vi "Test Panel - Sample (SubVI).vi"(8 "error in":errorcluster) -> (0 "error out":errorcluster, 3 "Data Out":T1)   [LabVIEW 2019]
uses:
  Controls/Sample-state.ctl
  <vilib>/httpClient/POSTBuffer.vi
  <vilib>/httpClient/LabVIEWHTTPClient.lvlib
panel:
  in  "Select Specimen From the list:":u16(ring) items=["Please Select..", "1 | 1", "2 | 2", "3 | 3", "4 | 4"]
  in  "Add/Remove Speciment":bool
  in  "Select Existing Job From the list:":u16(ring) items=["Please Select", "Job-001", "Job-002", "Job-003", "10125", "110125", "130125", "MB2695,S2"]
  in  "Refresh Button":bool
  in  "TAB":enum32{"Specimen Details"}(tab)
  in  "Close":bool
  in  "save":bool
  in  "table specimen":string[][](table)
  out "Table job record":string[][](table)
  in  "create new":bool
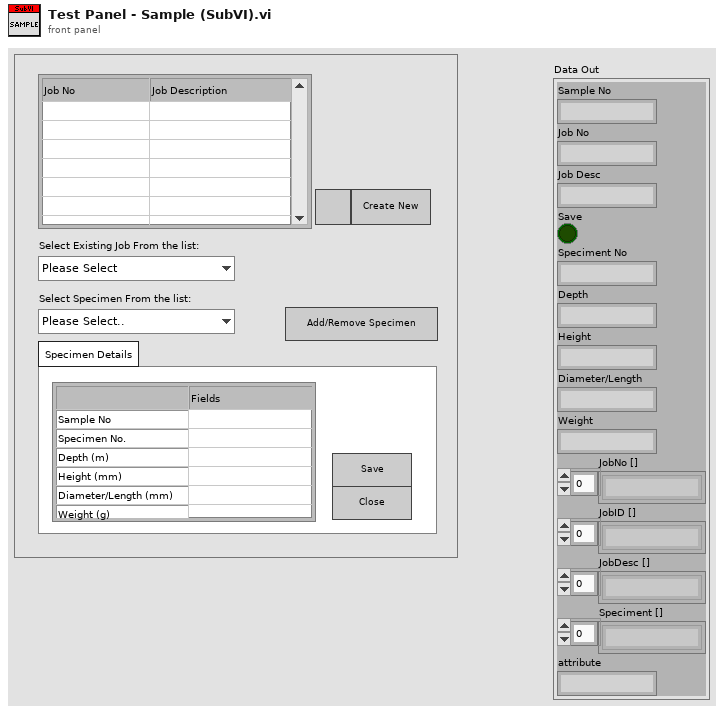
[diagram p1: front panel]
types:
  T1 = cluster{"Sample No":string, "Job No":string, "Job Desc":string, "Save":bool, "Speciment No":string, "Depth":string, "Height":string, "Diameter/Length":string, "Weight":string, "JobNo []":string[], "JobID []":string[], "JobDesc []":string[], "Speciment []":string[], "attribute":string}
  T2 = typedef "Sample-state.ctl" = enum16{"Init", "Read Config", "Idle", "Check", "Specimen", "Update", "Close"}
  T3 = cluster{"status":string, "data":cluster{"id":string, "jobno":string, "jobdesc":string, "delete":string}[]}
  T4 = cluster{"status":string, "data":cluster{"jobid":string, "sampleno":string, "specimentno":string, "weight":string, "height":string, "depth":string, "diameter":string, "delete":string, "id":string}[]}
  T5 = cluster{"status":string, "data":cluster{"jobid":string, "sampleno":string, "specimentno":string, "weight":string, "height":string, "depth":string, "diameter":string, "delete":string, "id":string, "attribute":string}[]}
  T6 = cluster{"Jobs No":string, "Key Value":string[]}[]
  T7 = typedef "LabVIEWHTTPClient.lvlib/ClientHandle.ctl" = refnum<k1>
  T8 = cluster{"id":string, "jobno":string, "jobdesc":string, "delete":string}[]
  T9 = cluster{"jobid":string, "sampleno":string, "specimentno":string, "weight":string, "height":string, "depth":string, "diameter":string, "delete":string, "id":string}[]
  T10 = cluster{"jobid":string, "sampleno":string, "specimentno":string, "weight":string, "height":string, "depth":string, "diameter":string, "delete":string, "id":string, "attribute":string}[]
  T11 = cluster{"jobid":string, "sampleno":string, "specimentno":string, "weight":string, "height":string, "depth":string, "diameter":string, "delete":string, "id":string, "attribute":string}
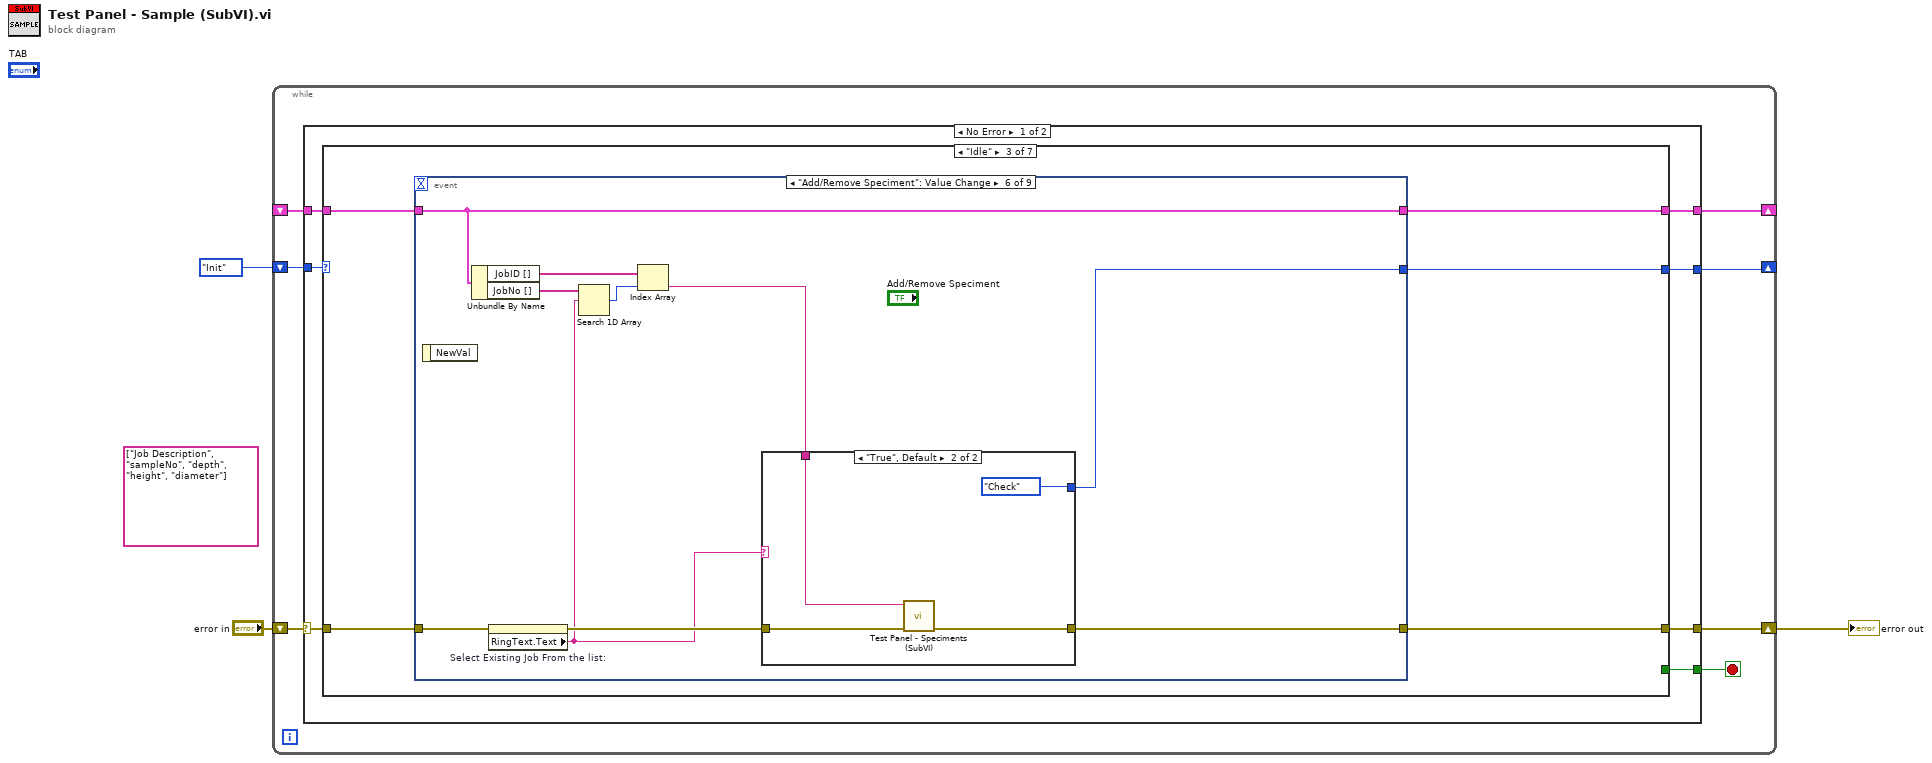
[diagram p0: block diagram]
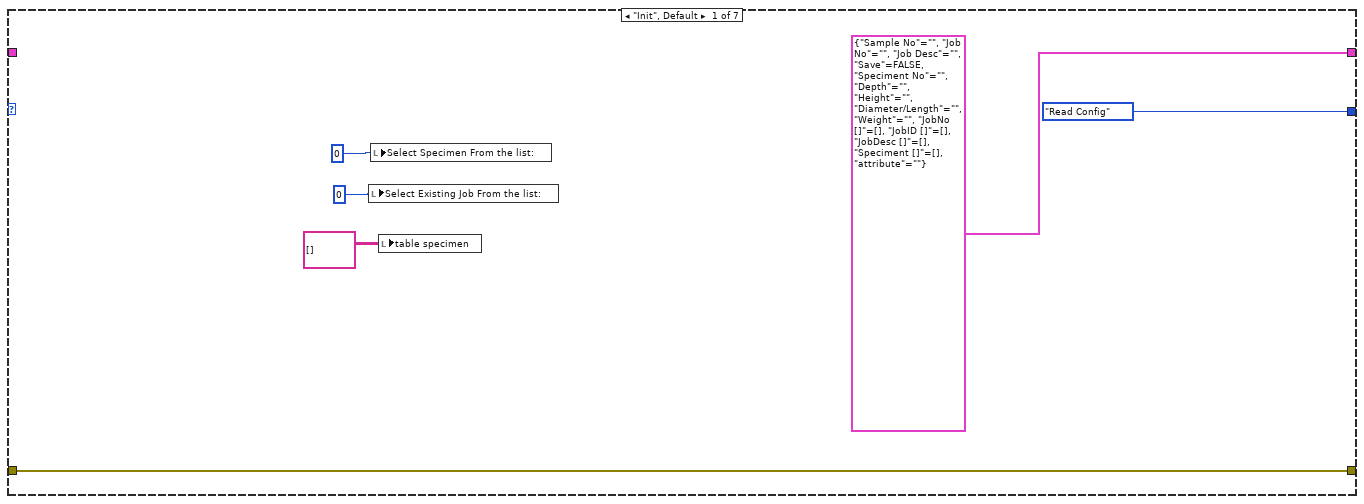
[diagram p2: hidden frame]
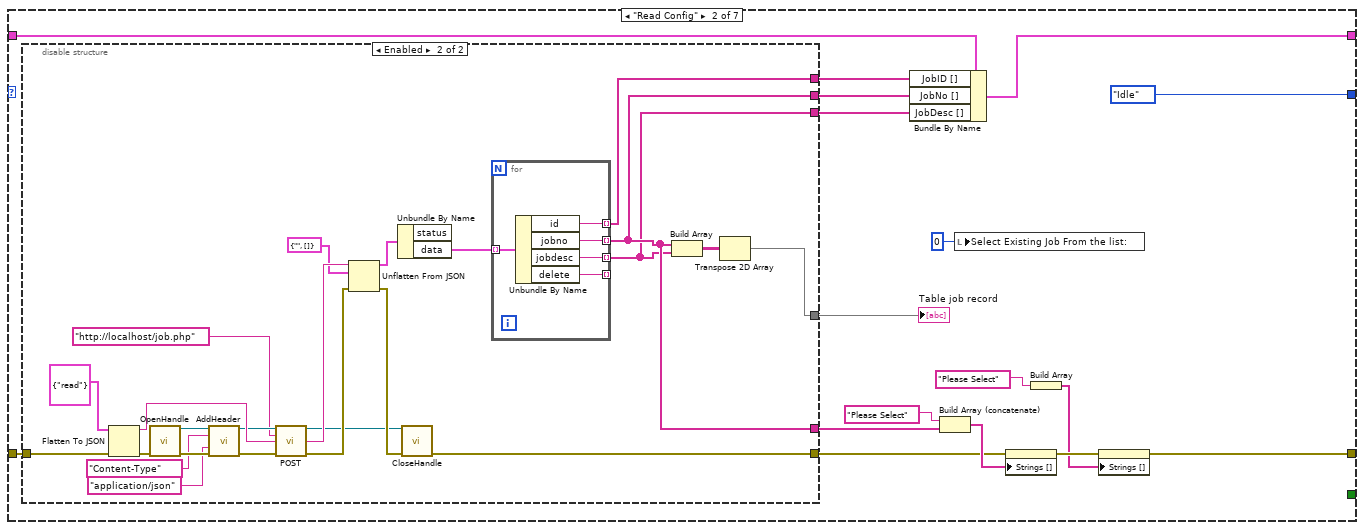
[diagram p3: hidden frame]
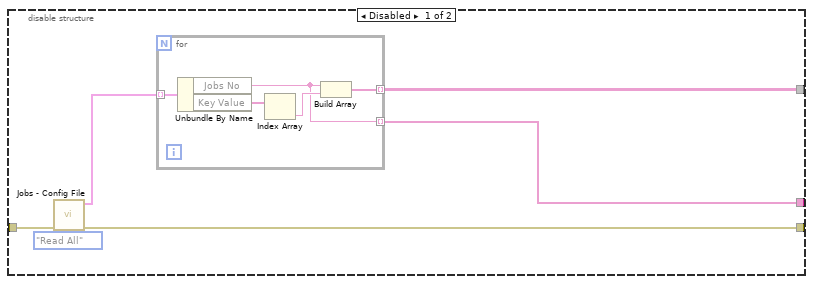
[diagram p4: hidden frame]
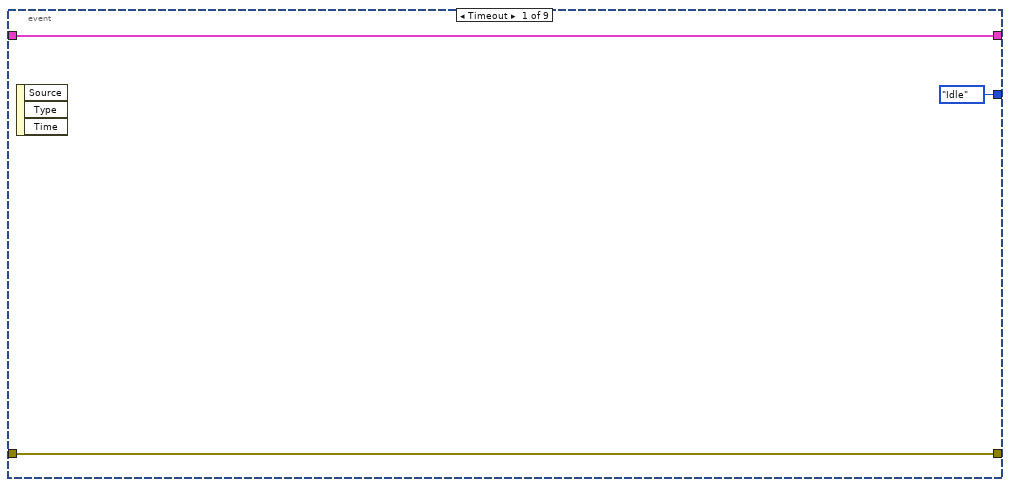
[diagram p5: hidden frame]
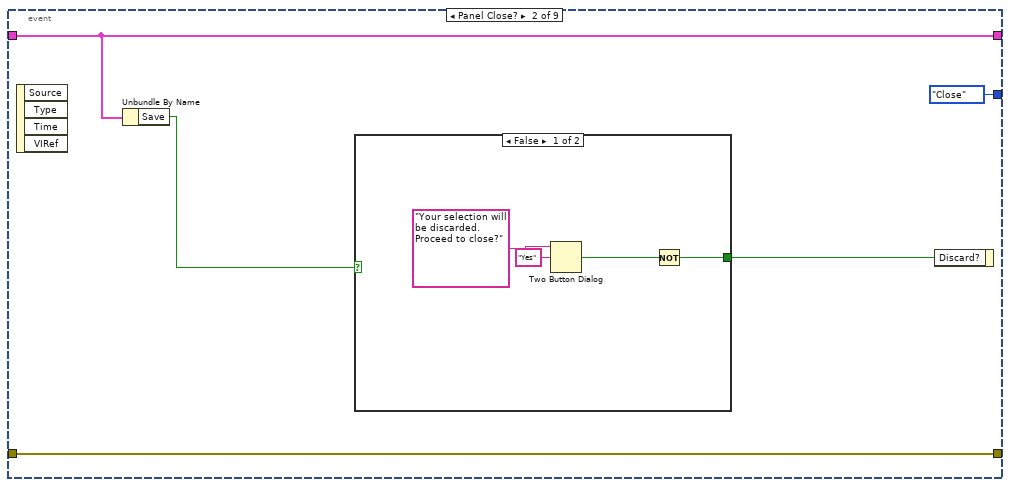
[diagram p6: hidden frame]
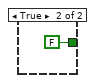
[diagram p7: hidden frame]
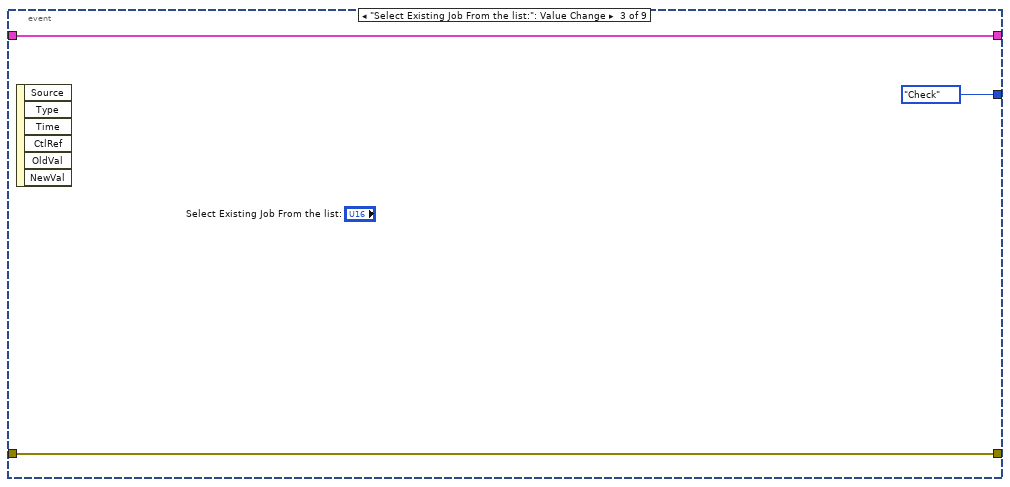
[diagram p8: hidden frame]
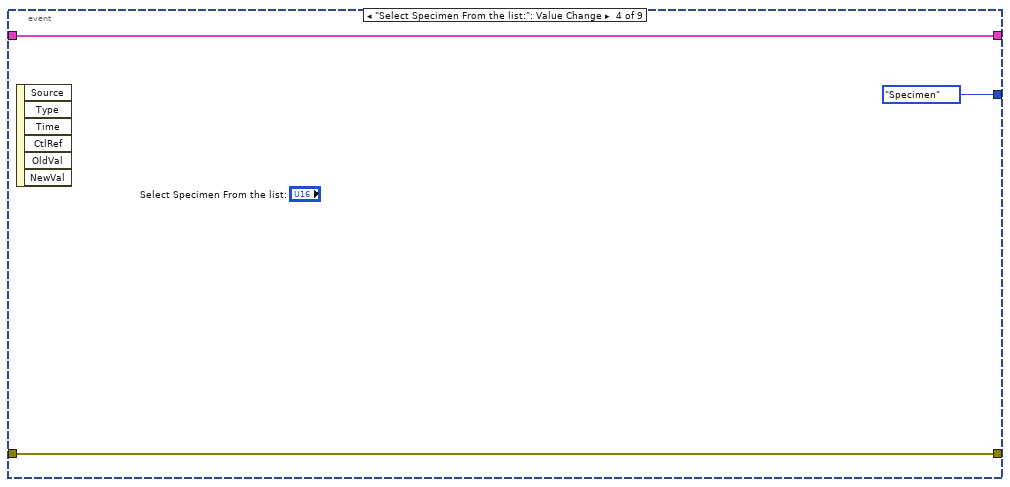
[diagram p9: hidden frame]
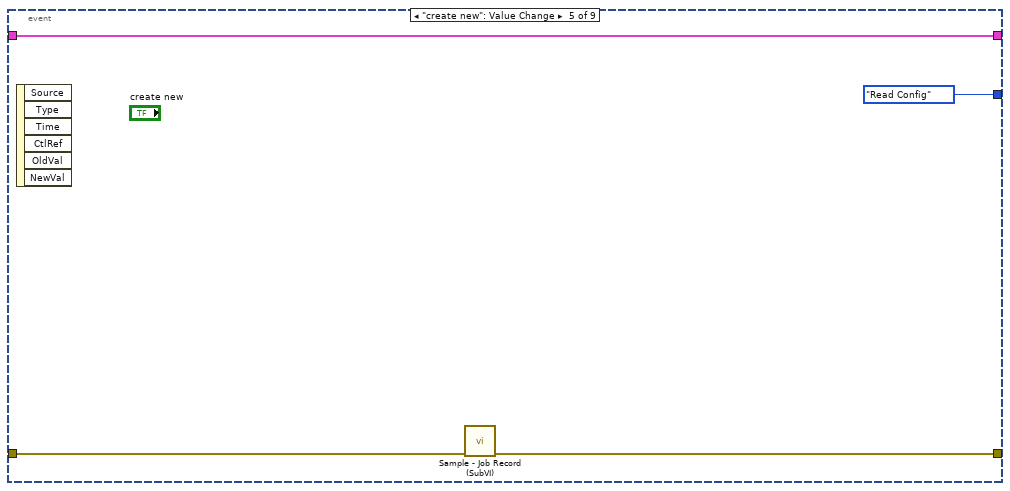
[diagram p10: hidden frame]
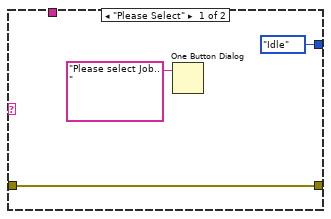
[diagram p11: hidden frame]
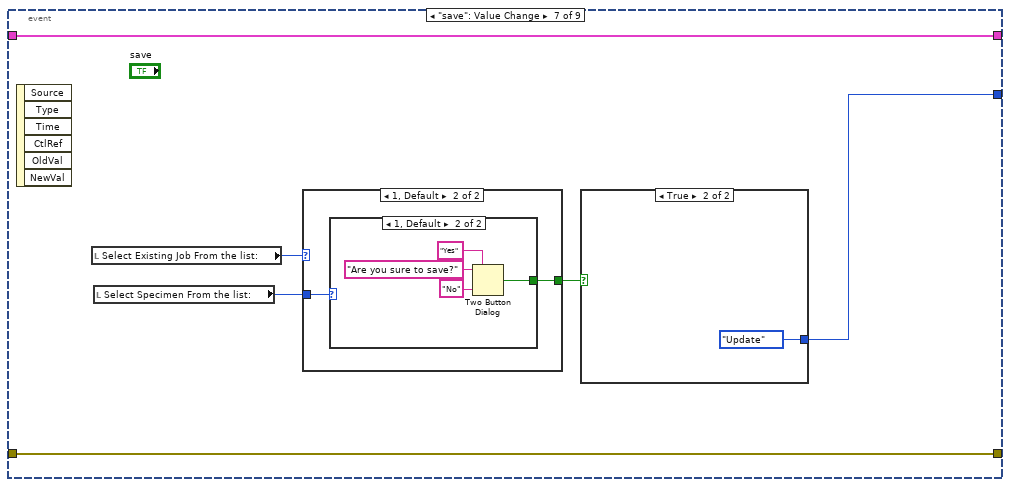
[diagram p12: hidden frame]
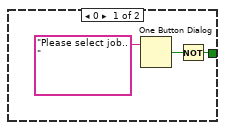
[diagram p13: hidden frame]
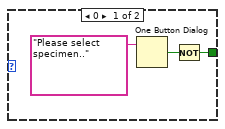
[diagram p14: hidden frame]
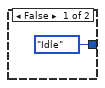
[diagram p15: hidden frame]
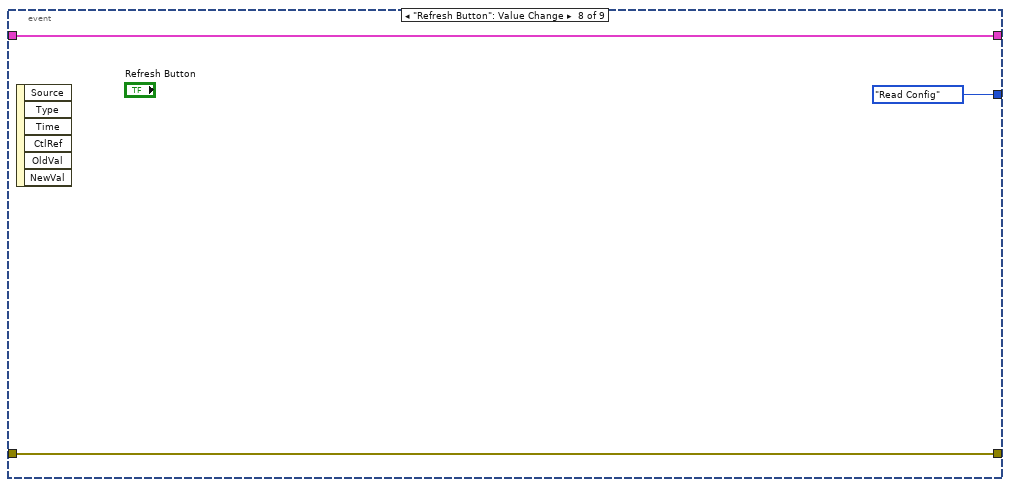
[diagram p16: hidden frame]
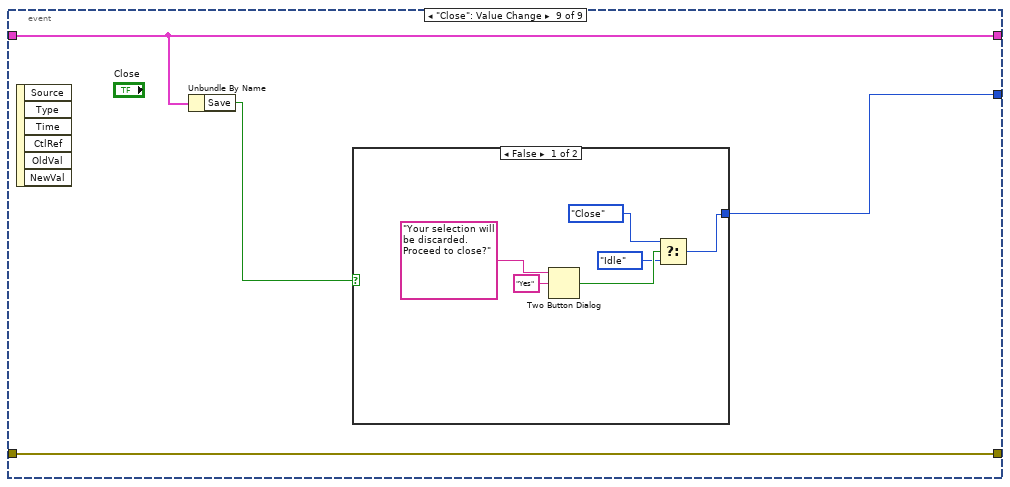
[diagram p17: hidden frame]
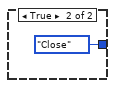
[diagram p18: hidden frame]
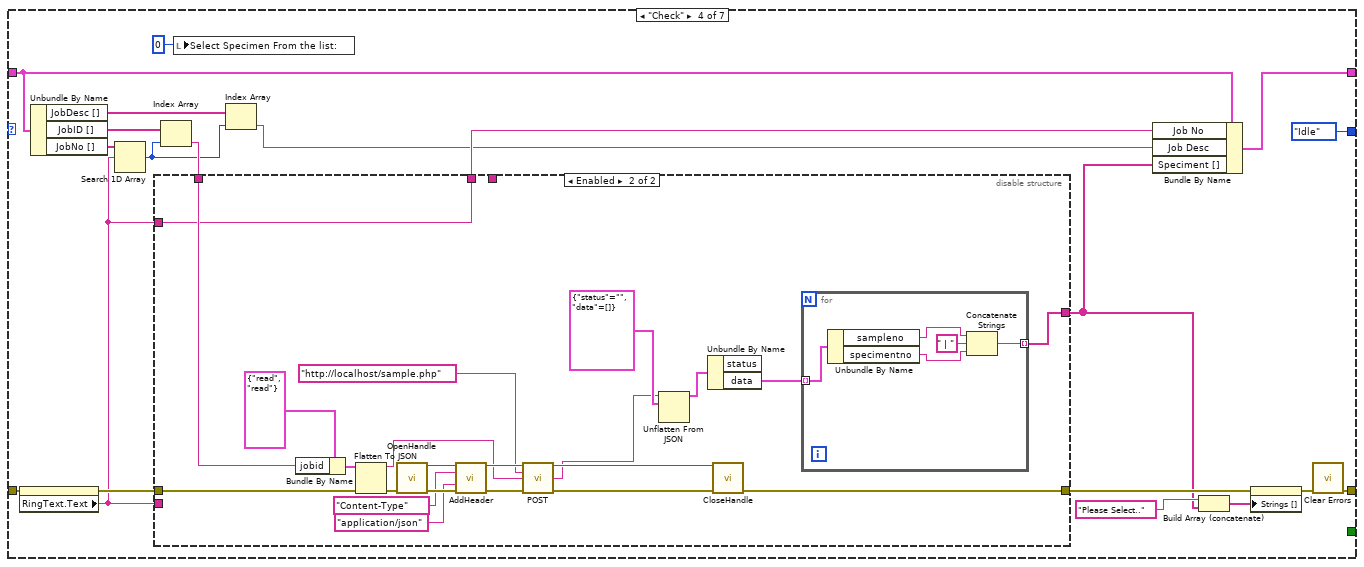
[diagram p19: hidden frame]
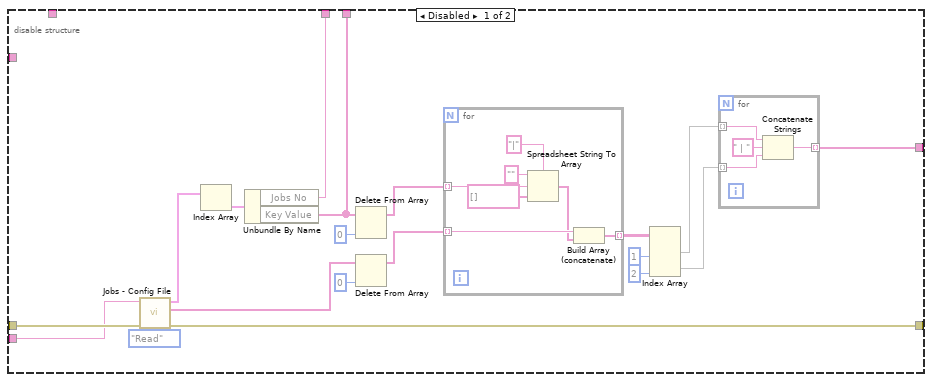
[diagram p20: hidden frame]
diagram:
  (unwired) string[] ["Job Description", "sampleNo", "depth", "height", "diameter"] ("Key Name")
  n1 = while {
    shift-right: [w8] -> w1
    shift-left: "error in" -> [w10]
    shift-right: [w7] -> _
    shift-left: Sample-state."Init" -> [w9]
    shift-right: [w6] -> _
    shift-left: _ -> [w5]
    stop <- w4 stop-if-true
    n2 = case shown="No Error" w10 {
      selector: w10 -> [w16 w356]
      tunnel: w9 -> [w17 _]
      tunnel: [w15 w355] -> w8
      tunnel: [w14 Sample-state."Idle"] -> w7
      tunnel: [w13 w353] -> w6
      tunnel: w5 -> [w12 w353]
      tunnel: [w11 _] -> w4
      frame No Error {
        n3 = case shown="\"Idle\"" w17 {
          tunnel: w16 -> [w20 w36 w85 w179 w262 w333 w351]
          tunnel: [w20 w31 w84 w178 w261 w331 w351] -> w15
          tunnel: [Sample-state."Read Config" Sample-state."Idle" w83 Sample-state."Idle" w253 w330 Sample-state."Close"] -> w14
          tunnel: [T1 {"Sample No"="", "Job No"="", "Job Desc"="", "Save"=FALSE, "Speciment No"="", "Depth"="", "Height"="", "Diameter/Length"="", "Weight"="", "JobNo []"=[], "JobID []"=[], "JobDesc []"=[], "Speciment []"=[], "attribute"=""} w28 w81 w175 w257 w328 T1 {"Sample No"="", "Job No"="", "Job Desc"="", "Save"=FALSE, "Speciment No"="", "Depth"="", "Height"="", "Diameter/Length"="", "Weight"="", "JobNo []"=[], "JobID []"=[], "JobDesc []"=[], "Speciment []"=[], "attribute"=""} ("Data Out")] -> w13
          tunnel: w12 -> [_ w27 w82 w168 w241 w327 w348]
          tunnel: [_ _ _ _ _ _ TRUE] -> w11
          frame "Init", Default {
            n4 = local write "Select Existing Job From the list:"(0) -> ()
            n5 = local write "Select Specimen From the list:"(0) -> ()
            n6 = local write "table specimen"(string[][] []) -> ()
          }
          frame "Read Config" {
            n7 = disable-structure shown="Enabled" {
              disable-tunnel: w36 -> [w45 w57]
              disable-tunnel: [w44 w55] -> w35
              disable-tunnel: [w42 w56] -> w34
              disable-tunnel: [w41 w53] -> w33
              disable-tunnel: [_ w54] -> w26
              disable-tunnel: [_ w53] -> w25
              disable-tunnel: [_ w52] -> w24
              frame Disabled {
                n8 = call "Jobs - Config File.vi"("Action"=enum16{"Write", "Read", "Read All", "Remove"}."Read All", "error in (no error)"=w45) -> ("error out"=w44:errorcluster, "Value Out"=w43:T6)  [unwired: 7 in, 1 out]
                n9 = for {
                  tunnel: w43 -> [w51] mode=indexing
                  tunnel: [w48] -> w42 mode=indexing
                  tunnel: [w47] -> w41 mode=indexing
                  n10 = Unbundle By Name(w51) -> ("Jobs No"=w47:string, "Key Value"=w50:string[])
                  n11 = Index Array(array=w50) -> (element=w49:string)  [unwired: 1 in]
                  n12 = Build Array(w47, w49) -> (w48:string[])
                }
              }
              frame Enabled {
                n13 = Flatten To JSON(anything=cluster{"action":string} {"action"="read"}, error in (no error)=w57) -> (JSON string=w69:string, 11:w68:errorcluster)  [unwired: 1 in]
                n14 = call <vilib>:"OpenHandle.vi"("error in (no error)"=w68) -> ("client handle out"=w65:T7, "error out"=w63:errorcluster)  [unwired: 13 in]
                n15 = call <vilib>:"AddHeader.vi"("client handle"=w65, "header"="Content-Type", "value"="application/json", "error in (no error)"=w63) -> ("client handle out"=w66:T7, "error out"=w64:errorcluster)  [unwired: 10 in]
                n16 = call-poly <vilib>:"POST.vi"("client handle"=w66, "url"="http://localhost/job.php", "buffer"=w69, "error in (no error)"=w64) -> ("client handle out"=w67:T7, "body"=w72:string, "error out"=w73:errorcluster)  [unwired: 8 in, 1 out]
                n17 = Unflatten From JSON(JSON string=w72, type and defaults=T3 {"status"="", "data"=[]}, error in (no error)=w73) -> (value=w70:T3, error out=w74:errorcluster)  [unwired: 4 in]
                n18 = Unbundle By Name(w70) -> ("data"=w71:T8)  [unwired: 1 out]
                n19 = call <vilib>:"CloseHandle.vi"("client handle"=w67, "error in (no error)"=w74) -> ("error out"=w55:errorcluster)  [unwired: 13 in]
                n20 = for {
                  tunnel: w71 -> [w80] mode=indexing
                  tunnel: [w79] -> w54 mode=indexing
                  tunnel: [w78] -> w53 mode=indexing
                  tunnel: [w77] -> w52 mode=indexing
                  tunnel: [w76] -> _ mode=indexing
                  n21 = Unbundle By Name(w80) -> ("id"=w79:string, "jobno"=w78:string, "jobdesc"=w77:string, "delete"=w76:string)
                }
                n22 = Build Array(w53, w52) -> (w75:string[][])
                n23 = Transpose 2D Array(2D array=w75) -> (transposed array=w56:string[][])
              }
            }
            "Table job record" <- w34
            n24 = Bundle By Name(cluster=w27, "JobID []"=w26, "JobNo []"=w25, "JobDesc []"=w24) -> (w28:T1)
            n25 = Build Array (concatenate)("Please Select", w33) -> (w38:string[])
            n26 = local write "Select Existing Job From the list:"(0) -> ()
            n27 = property on="Select Existing Job From the list:" class="Ring (strict)"(error in=w35, "Strings []"=w38) -> (error out=w32:errorcluster)  [unwired: 1 in, 1 out]
            n28 = Build Array("Please Select") -> (w29:string[])
            n29 = property on="Select Specimen From the list:" class="Ring (strict)"(error in=w32, "Strings []"=w29) -> (error out=w31:errorcluster)  [unwired: 1 in, 1 out]
          }
          frame "Idle" {
            n30 = event shown="[5] \"Add/Remove Speciment\": Value Change" {
              selector: _ -> [_ _ _ _ _ _ _ _ _]
              dyn-events: _ -> [_ _ _ _ _ _ _ _ _]
              timeout: _ -> [_ _ _ _ _ _ _ _ _]
              tunnel: w85 -> [w88 w93 w99 w102 w105 w116 w129 w147 w152]
              tunnel: [w88 w93 w99 w102 w106 w118 w129 w147 w152] -> w84
              tunnel: [Sample-state."Idle" Sample-state."Close" Sample-state."Check" Sample-state."Specimen" Sample-state."Read Config" w115 w130 Sample-state."Read Config" w149] -> w83
              tunnel: w82 -> [w86 w91 w101 w104 w107 w114 w128 w146 w151]
              tunnel: [w86 w91 w101 w104 w107 w114 w128 w146 w151] -> w81
              event Timeout {
                n31 = event-data() -> ()  [unwired: 1 in, 3 out]
              }
              event Panel Close? {
                n32 = event-data() -> ()  [unwired: 1 in, 4 out]
                n33 = Unbundle By Name(w91) -> ("Save"=w90:bool)
                n34 = case shown="False" w90 {
                  tunnel: [w95 FALSE] -> w89
                  frame False {
                    n35 = Two Button Dialog(message="Your selection will be discarded. Proceed to close?", 2:"Yes" ("T button name (\"OK\")")) -> (T button?=w96:bool)  [unwired: 1 in]
                    n36 = Not(x=w96) -> (.not. x?=w95:bool)
                  }
                  frame True {
                  }
                }
                n37 = event-data("Discard?"=w89) -> ()  [unwired: 1 in, 1 out]
              }
              event "Select Existing Job From the list:": Value Change {
                n38 = event-data() -> ()  [unwired: 1 in, 6 out]
              }
              event "Select Specimen From the list:": Value Change {
                n39 = event-data() -> ()  [unwired: 1 in, 6 out]
              }
              event "create new": Value Change {
                n40 = event-data() -> ()  [unwired: 1 in, 6 out]
                n41 = call "Sample - Job Record (SubVI).vi"("error in"=w105) -> ("error out"=w106:errorcluster)  [unwired: 10 in]
              }
              event "Add/Remove Speciment": Value Change {
                n42 = event-data() -> ()  [unwired: 1 in, 1 out]
                n43 = Unbundle By Name(w114) -> ("JobID []"=w111:string[], "JobNo []"=w113:string[])
                n44 = property on="Select Existing Job From the list:" class="Ring (strict)"(error in=w116) -> (error out=w117:errorcluster, "RingText.Text"=w112:string)  [unwired: 1 in, 1 out]
                n45 = Search 1D Array(1D array=w113, element=w112) -> (index of element=w110:i32)  [unwired: 1 in]
                n46 = Index Array(array=w111, index=w110) -> (element=w109:string)
                n47 = case shown="\"True\", Default" w112 {
                  tunnel: [w121 w125] -> w118
                  tunnel: w117 -> [w121 w124]
                  tunnel: [Sample-state."Idle" Sample-state."Check"] -> w115
                  tunnel: w109 -> [_ w122]
                  frame "Please Select" {
                    n48 = One Button Dialog(message="Please select Job..") -> ()  [unwired: 1 in, 1 out]
                  }
                  frame "True", Default {
                    n49 = call "Test Panel - Speciments (SubVI).vi"("error in"=w124, "Job ID"=w122) -> ("error out"=w125:errorcluster)  [unwired: 9 in]
                  }
                }
              }
              event "save": Value Change {
                n50 = event-data() -> ()  [unwired: 1 in, 6 out]
                n51 = local read "Select Existing Job From the list:"() -> (w127:u16)
                n52 = local read "Select Specimen From the list:"() -> (w126:u16)
                n53 = case shown="1, Default" w127 {
                  tunnel: [w132 w136] -> w131
                  tunnel: w126 -> [_ w135]
                  frame 0 {
                    n54 = One Button Dialog(message="Please select job..") -> (true=w133:bool)  [unwired: 1 in]
                    n55 = Not(x=w133) -> (.not. x?=w132:bool)
                  }
                  frame 1, Default {
                    n56 = case shown="1, Default" w135 {
                      tunnel: [w137 w140] -> w136
                      frame 0 {
                        n57 = One Button Dialog(message="Please select specimen..") -> (true=w138:bool)  [unwired: 1 in]
                        n58 = Not(x=w138) -> (.not. x?=w137:bool)
                      }
                      frame 1, Default {
                        n59 = Two Button Dialog(message="Are you sure to save?", 1:"No" ("F button name (\"Cancel\")"), 2:"Yes" ("T button name (\"OK\")")) -> (T button?=w140:bool)
                      }
                    }
                  }
                }
                n60 = case shown="True" w131 {
                  tunnel: [Sample-state."Idle" Sample-state."Update"] -> w130
                  frame False {
                  }
                  frame True {
                  }
                }
              }
              event "Refresh Button": Value Change {
                n61 = event-data() -> ()  [unwired: 1 in, 6 out]
              }
              event "Close": Value Change {
                n62 = event-data() -> ()  [unwired: 1 in, 6 out]
                n63 = Unbundle By Name(w151) -> ("Save"=w150:bool)
                n64 = case shown="False" w150 {
                  tunnel: [w155 Sample-state."Close" ("f")] -> w149
                  frame False {
                    n65 = Two Button Dialog(message="Your selection will be discarded. Proceed to close?", 2:"Yes" ("T button name (\"OK\")")) -> (T button?=w157:bool)  [unwired: 1 in]
                    n66 = Select(t=Sample-state."Close", s=w157, f=Sample-state."Idle") -> (s? t:f=w155:T2)
                  }
                  frame True {
                  }
                }
              }
            }
          }
          frame "Check" {
            n67 = property on="Select Existing Job From the list:" class="Ring (strict)"(error in=w179) -> (error out=w177:errorcluster, "RingText.Text"=w164:string)  [unwired: 1 in, 1 out]
            n68 = Unbundle By Name(w168) -> ("JobDesc []"=w163:string[], "JobID []"=w166:string[], "JobNo []"=w167:string[])
            n69 = Search 1D Array(1D array=w167, element=w164) -> (index of element=w162:i32)  [unwired: 1 in]
            n70 = Index Array(array=w166, index=w162) -> (element=w165:string)
            n71 = disable-structure shown="Enabled" {
              disable-tunnel: w177 -> [w197 w216]
              disable-tunnel: [w193 w210] -> w176
              disable-tunnel: [w192 _] -> _
              disable-tunnel: [w185 w215] -> w173
              disable-tunnel: [w181 w211] -> w160
              disable-tunnel: w164 -> [w180 _]
              disable-tunnel: w165 -> [_ w214]
              disable-tunnel: w164 -> [_ w210]
              frame Disabled {
                n72 = call "Jobs - Config File.vi"("Action"=enum16{"Write", "Read", "Read All", "Remove"}."Read", "error in (no error)"=w197, "Jobs No"=w180) -> ("error out"=w185:errorcluster, "key names"=w189:string[], "Value Out"=w196:T6)  [unwired: 6 in]
                n73 = Index Array(array=w196) -> (element=w195:cluster{"Jobs No":string, "Key Value":string[]})  [unwired: 1 in]
                n74 = Unbundle By Name(w195) -> ("Jobs No"=w193:string, "Key Value"=w192:string[])
                n75 = Delete From Array(array=w192, index=0) -> (array with subset deleted=w191:string[])  [unwired: 1 in, 1 out]
                n76 = Delete From Array(array=w189, index=0) -> (array with subset deleted=w188:string[])  [unwired: 1 in, 1 out]
                n77 = for {
                  tunnel: w188 -> [w205] mode=indexing
                  tunnel: w191 -> [w209] mode=indexing
                  tunnel: [w203] -> w187 mode=indexing
                  n78 = Spreadsheet String To Array(delimiter (Tab)="|", format string="", spreadsheet string=w209, array type (2D Dbl)=string[] []) -> (array=w204:string[])
                  n79 = Build Array (concatenate)(w205, w204) -> (w203:string[])
                }
                n80 = Index Array(array=w187, index (col) #1=1 ("disabled index (col)"), index (col) #2=2 ("index (col)")) -> (element #1=w183:string[], element #2=w182:string[])  [unwired: 2 in]
                n81 = for {
                  tunnel: w183 -> [w202] mode=indexing
                  tunnel: w182 -> [w201] mode=indexing
                  tunnel: [w199] -> w181 mode=indexing
                  n82 = Concatenate Strings(w202, " | " ("string"), w201) -> (w199:string)
                }
              }
              frame Enabled {
                n83 = Bundle By Name(cluster=cluster{"action":string, "jobid":string} {"action"="read", "jobid"="read"}, "jobid"=w214) -> (w212:cluster{"action":string, "jobid":string})
                n84 = Flatten To JSON(anything=w212, error in (no error)=w216) -> (JSON string=w224:string, 11:w225:errorcluster)  [unwired: 1 in]
                n85 = call <vilib>:"OpenHandle.vi"("error in (no error)"=w225) -> ("client handle out"=w229:T7, "error out"=w231:errorcluster)  [unwired: 13 in]
                n86 = call <vilib>:"AddHeader.vi"("client handle"=w229, "header"="Content-Type", "value"="application/json", "error in (no error)"=w231) -> ("client handle out"=w228:T7, "error out"=w230:errorcluster)  [unwired: 10 in]
                n87 = call-poly <vilib>:"POST.vi"("client handle"=w228, "url"="http://localhost/sample.php", "buffer"=w224, "error in (no error)"=w230) -> ("client handle out"=w226:T7, "body"=w217:string, "error out"=w227:errorcluster)  [unwired: 8 in, 1 out]
                n88 = Unflatten From JSON(JSON string=w217, type and defaults=T4 {"status"="", "data"=[]}) -> (value=w219:T4)  [unwired: 5 in, 1 out]
                n89 = Unbundle By Name(w219) -> ("data"=w218:T9)  [unwired: 1 out]
                n90 = call <vilib>:"CloseHandle.vi"("client handle"=w226, "error in (no error)"=w227) -> ("error out"=w215:errorcluster)  [unwired: 13 in]
                n91 = for {
                  tunnel: w218 -> [w236] mode=indexing
                  tunnel: [w232] -> w211 mode=indexing
                  n92 = Unbundle By Name(w236) -> ("sampleno"=w234:string, "specimentno"=w233:string)
                  n93 = Concatenate Strings(w234, " | " ("string"), w233) -> (w232:string)
                }
              }
            }
            n94 = local write "Select Specimen From the list:"(0) -> ()
            n95 = Index Array(array=w163, index=w162) -> (element=w161:string)
            n96 = Bundle By Name(cluster=w168, "Job No"=w176, "Job Desc"=w161, "Speciment []"=w160) -> (w175:T1)
            n97 = Build Array (concatenate)("Please Select..", w160) -> (w171:string[])
            n98 = property on="Select Specimen From the list:" class="Ring (strict)"(error in=w173, "Strings []"=w171) -> (error out=w172:errorcluster)  [unwired: 1 in, 1 out]
            n99 = call <vilib>:"Clear Errors.vi"("error in (no error)"=w172) -> ("error out"=w178:errorcluster)  [unwired: 5 in, 1 out]
          }
          frame "Specimen" {
            n100 = property on="Select Existing Job From the list:" class="Ring (strict)"(error in=w262) -> (error out=w260:errorcluster, "RingText.Text"=w240:string)  [unwired: 1 in, 1 out]
            n101 = Unbundle By Name(w241) -> ("Speciment []"=w238:string[], "JobID []"=w243:string[], "JobNo []"=w244:string[])
            n102 = Search 1D Array(1D array=w244, element=w240) -> (index of element=w242:i32)  [unwired: 1 in]
            n103 = Index Array(array=w243, index=w242) -> (element=w239:string)
            n104 = disable-structure shown="Enabled" {
              disable-tunnel: w260 -> [w285 w307]
              disable-tunnel: w240 -> [w284 _]
              disable-tunnel: [w275 w309] -> w252
              disable-tunnel: [w269 w295] -> w251
              disable-tunnel: [w268 w301] -> w250
              disable-tunnel: [w267 w300] -> w249
              disable-tunnel: [w266 w299] -> w248
              disable-tunnel: [w265 w298] -> w247
              disable-tunnel: [w264 w297] -> w246
              disable-tunnel: [w263 w296] -> w245
              disable-tunnel: w239 -> [_ w310]
              disable-tunnel: w238 -> [_ w304]
              disable-tunnel: [_ w294] -> w237
              frame Disabled {
                n105 = call "Jobs - Config File.vi"("Action"=enum16{"Write", "Read", "Read All", "Remove"}."Read", "error in (no error)"=w285, "Jobs No"=w284) -> ("error out"=w275:errorcluster, "key names"=w277:string[], "Value Out"=w283:T6)  [unwired: 6 in]
                n106 = Index Array(array=w283) -> (element=w282:cluster{"Jobs No":string, "Key Value":string[]})  [unwired: 1 in]
                n107 = Unbundle By Name(w282) -> ("Key Value"=w280:string[])
                n108 = Delete From Array(array=w280, index=0) -> (array with subset deleted=w279:string[])  [unwired: 1 in, 1 out]
                n109 = Delete From Array(array=w277, index=0) -> (array with subset deleted=w276:string[])  [unwired: 1 in, 1 out]
                n110 = local read "Select Specimen From the list:"() -> (w271:u16)
                n111 = for {
                  tunnel: w276 -> [w289] mode=indexing
                  tunnel: w279 -> [w293] mode=indexing
                  tunnel: [w287] -> w274 mode=indexing
                  n112 = Spreadsheet String To Array(delimiter (Tab)="|", format string="", spreadsheet string=w293, array type (2D Dbl)=string[] []) -> (array=w288:string[])
                  n113 = Build Array (concatenate)(w289, w288) -> (w287:string[])
                }
                n114 = Decrement(x=w271) -> (x-1=w270:u16)
                n115 = Delete From Array(array=w274, index (col)=0 ("disabled index (col)")) -> (array with subset deleted=w273:string[][])  [unwired: 2 in, 1 out]
                n116 = Index Array(array=w273, index (row)=w270) -> (element=w269:string[])  [unwired: 1 in]
                n117 = Index Array(array=w269) -> (element #1=w268:string, element #2=w267:string, element #3=w266:string, element #4=w265:string, element #5=w264:string, element #6=w263:string)  [unwired: 6 in]
              }
              frame Enabled {
                n118 = property on="Select Specimen From the list:" class="Ring (strict)"(error in=w307) -> (error out=w308:errorcluster, "RingText.Text"=w305:string)  [unwired: 1 in, 1 out]
                n119 = Search 1D Array(1D array=w304, element=w305) -> (index of element=w303:i32)  [unwired: 1 in]
                n120 = Bundle By Name(cluster=cluster{"action":string, "jobid":string} {"action"="read", "jobid"="read"}, "jobid"=w310) -> (w311:cluster{"action":string, "jobid":string})
                n121 = Flatten To JSON(anything=w311, error in (no error)=w308) -> (JSON string=w319:string, 11:w320:errorcluster)  [unwired: 1 in]
                n122 = call <vilib>:"OpenHandle.vi"("error in (no error)"=w320) -> ("client handle out"=w324:T7, "error out"=w326:errorcluster)  [unwired: 13 in]
                n123 = call <vilib>:"AddHeader.vi"("client handle"=w324, "header"="Content-Type", "value"="application/json", "error in (no error)"=w326) -> ("client handle out"=w323:T7, "error out"=w325:errorcluster)  [unwired: 10 in]
                n124 = call-poly <vilib>:"POST.vi"("client handle"=w323, "url"="http://localhost/sample.php", "buffer"=w319, "error in (no error)"=w325) -> ("client handle out"=w321:T7, "body"=w313:string, "error out"=w322:errorcluster)  [unwired: 8 in, 1 out]
                n125 = Unflatten From JSON(JSON string=w313, type and defaults=T5 {"status"="", "data"=[]}) -> (value=w314:T5)  [unwired: 5 in, 1 out]
                n126 = Unbundle By Name(w314) -> ("data"=w306:T10)  [unwired: 1 out]
                n127 = call <vilib>:"CloseHandle.vi"("client handle"=w321, "error in (no error)"=w322) -> ("error out"=w309:errorcluster)  [unwired: 13 in]
                n128 = Index Array(array=w306, index=w303) -> (element=w302:T11)
                n129 = Unbundle By Name(w302) -> ("attribute"=w294:string, "sampleno"=w301:string, "specimentno"=w300:string, "depth"=w299:string, "height"=w298:string, "diameter"=w297:string, "weight"=w296:string)
                n130 = Build Array(w301, w300, w299, w298, w297, w296) -> (w295:string[])
              }
            }
            n131 = Bundle By Name(cluster=w241, "attribute"=w237, "Sample No"=w250, "Speciment No"=w249, "Depth"=w248, "Height"=w247, "Diameter/Length"=w246, "Weight"=w245) -> (w257:T1)
            n132 = Build Array(w251) -> (w259:string[][])
            n133 = Transpose 2D Array(2D array=w259) -> (transposed array=w258:string[][])
            n134 = Unbundle By Name(w257) -> ("Save"=w256:bool)
            n135 = local write "table specimen"(w258) -> ()
            n136 = Select(t=Sample-state."Close", s=w256, f=Sample-state."Idle") -> (s? t:f=w253:T2)
            n137 = call <vilib>:"Clear Errors.vi"("error in (no error)"=w252) -> ("error out"=w261:errorcluster)  [unwired: 5 in, 1 out]
          }
          frame "Update" {
            n138 = disable-structure shown="Disabled" {
              disable-tunnel: w333 -> [w341 w343]
              disable-tunnel: [w334 w343] -> w332
              frame Disabled {
                n139 = property on="Select Existing Job From the list:" class="Ring (strict)"(error in=w341) -> (error out=w340:errorcluster, "RingText.Text"=w339:string)  [unwired: 1 in, 1 out]
                n140 = Index Array(array="table specimen", index (col)=0 ("disabled index (col)")) -> (element=w335:string[])  [unwired: 1 in]
                n141 = call "Jobs - Config File.vi"("Action"=enum16{"Write", "Read", "Read All", "Remove"}."Write", "error in (no error)"=w340, "Value"=w335, "Key Name"=string[] ["sampleNo", "depth", "height", "diameter", "weight"], "Jobs No"=w339) -> ("error out"=w334:errorcluster)  [unwired: 4 in, 2 out]
              }
              frame Enabled {
              }
            }
            n142 = Bundle By Name(cluster=w327, "Save"=TRUE) -> (w328:T1)
            n143 = case shown="No Error" w332 {
              selector: w332 -> [w345 w347]
              tunnel: [w345 w347] -> w331
              tunnel: [Sample-state."Specimen" Sample-state."Idle"] -> w330
              frame No Error {
              }
              frame Error {
              }
            }
          }
          frame "Close" {
            "Data Out" <- w348
          }
        }
      }
      frame Error {
        n144 = call <vilib>:"Clear Errors.vi"("error in (no error)"=w356) -> ("error out"=w355:errorcluster)  [unwired: 5 in, 1 out]
      }
    }
  }
  "error out" <- w1
